vi "LIA Configure Decimators.vi"(5 "lock-in.decimator1 0":T1, 7 "lock-in.decimator0 0":T2, 8 "error in (no error)":errorcluster, 9 "lock-in.decimation1 0":i32, 10 "lock-in.decimation0 0":i32, 11 "LIA Host Interface in":refnum<class "LIA Host Interface.lvclass">) -> (0 "error out":errorcluster, 3 "LIA Host Interface out":refnum<class "LIA Host Interface.lvclass">)   [LabVIEW 2017]
uses:
  Program Files (x86)/National Instruments/LabVIEW 2017/examples/Lock-In Amplifier/lib/interface/Interface/LIA Host Interface.lvclass
  FPGA/LIA Decimator0 Enum.ctl
  FPGA/LIA Decimator1 Enum.ctl
  Program Files (x86)/National Instruments/LabVIEW 2017/examples/Lock-In Amplifier/lib/interface/Interface FPGA/LIA Host Interface FPGA.lvclass
  Program Files (x86)/National Instruments/LabVIEW 2017/examples/Lock-In Amplifier/lib/host/Public/fpga type.ctl
  Program Files (x86)/National Instruments/LabVIEW 2017/examples/Lock-In Amplifier/lib/interface/Interface FPGA/Properties/FpgaSession_GET.vi
  <vilib>/Utility/error.llb/Error Cluster From Error Code.vi
  <vilib>/rvi/errors/niLvFpgaAdjustHostInterfaceError.vi
  <vilib>/rvi/interface/nirviReadWriteControl/nirviReadWriteControl.xnode
  Program Files (x86)/National Instruments/LabVIEW 2017/examples/Lock-In Amplifier/lib/host/Lock-In Amplifier Example Host.lvlib
  NiFpgaLv.dll
  <vilib>/rvi/interface/Simulation/niFpgaSimulationCallBeginRW.vi
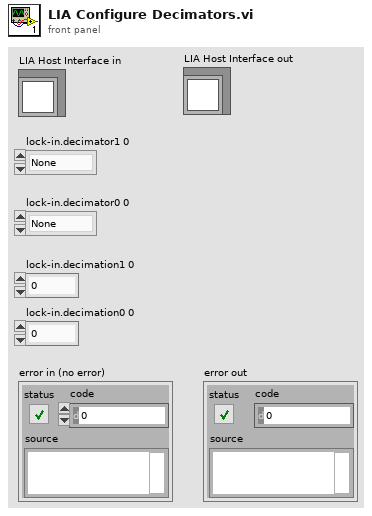
[diagram p1: front panel]
types:
  T1 = typedef "LIA Decimator1 Enum.ctl" = enum16{"None", "FIR", "SOS"}
  T2 = typedef "LIA Decimator0 Enum.ctl" = enum16{"None", "CIC", "FIR", "4HB", "SOS"}
  T3 = typedef "Lock-In Amplifier Example Host.lvlib/fpga type.ctl" = refnum<k20>
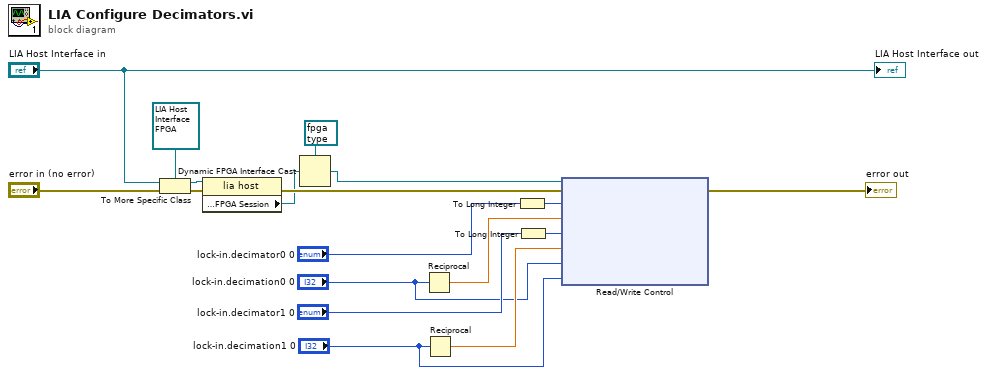
[diagram p0: block diagram]
diagram:
  n1 = To More Specific Class(target class=refnum<class "LIA Host Interface FPGA.lvclass"> refnum ("lia host"), reference="LIA Host Interface in", error in="error in (no error)") -> (specific class reference=w13:refnum<class "LIA Host Interface FPGA.lvclass">, error out=w12:errorcluster)
  n2 = property class="lia host"(reference=w13, error in=w12) -> (error out=w18:errorcluster, "Properties:FPGA Session"=w14:refnum<k20>)  [unwired: 1 out]
  n3 = Dynamic FPGA Interface Cast(Session In=T3 refnum ("fpga type"), Type=w14) -> (Session Out=w8:T3)
  n4 = Reciprocal(x="lock-in.decimation0 0") -> (1/x=w17:dbl)
  n5 = Reciprocal(x="lock-in.decimation1 0") -> (1/x=w6:dbl)
  n6 = To Long Integer(number="lock-in.decimator0 0") -> (32bit integer=w4:i32)
  n7 = To Long Integer(number="lock-in.decimator1 0") -> (32bit integer=w3:i32)
  n8 = xnode "Read/Write Control"("FPGA VI Reference In"=w8, "error in"=w18, "lock-in.decimator0 0"=w4, "lock-in.fir0 fs 0"=w17, "lock-in.decimator1 0"=w3, "lock-in.fir1 fs 0"=w6, "lock-in.iir decimation0 0"="lock-in.decimation0 0", "lock-in.iir decimation1 0"="lock-in.decimation1 0") -> ("error out"=→"error out":errorcluster)  [unwired: 1 out]
  "LIA Host Interface out" <- "LIA Host Interface in"
